vi "poly_diff_I32.vi"(2 "input":i32[](array[numeric])) -> (7 "output":i32[](array[numeric]))   [LabVIEW 2015]
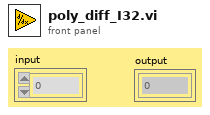
[diagram p1: front panel]
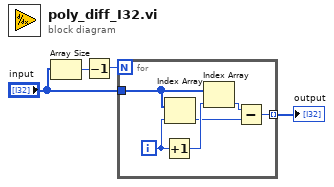
[diagram p0: block diagram]
diagram:
  n1 = Array Size(array="input") -> (size(s)=w3:i32)
  n2 = Decrement(x=w3) -> (x-1=w2:i32)
  n3 = for {
    N: w2 -> [_]
    tunnel: "input" -> [w8]
    tunnel: [w5] -> w1 mode=indexing
    i -> [w9]
    n4 = Increment(x=w9) -> (x+1=w10:i32)
    n5 = Index Array(array=w8, index=w9) -> (element=w6:i32)
    n6 = Index Array(array=w8, index=w10) -> (element=w7:i32)
    n7 = Subtract(x=w7, y=w6) -> (x-y=w5:i32)
  }
  "output" <- w1
